vi "输入读取.vi"() -> (3 "输入读取":T1)   [LabVIEW 2017]
panel:
  in  "屏蔽光栅":bool
  out "运行时间":dbl
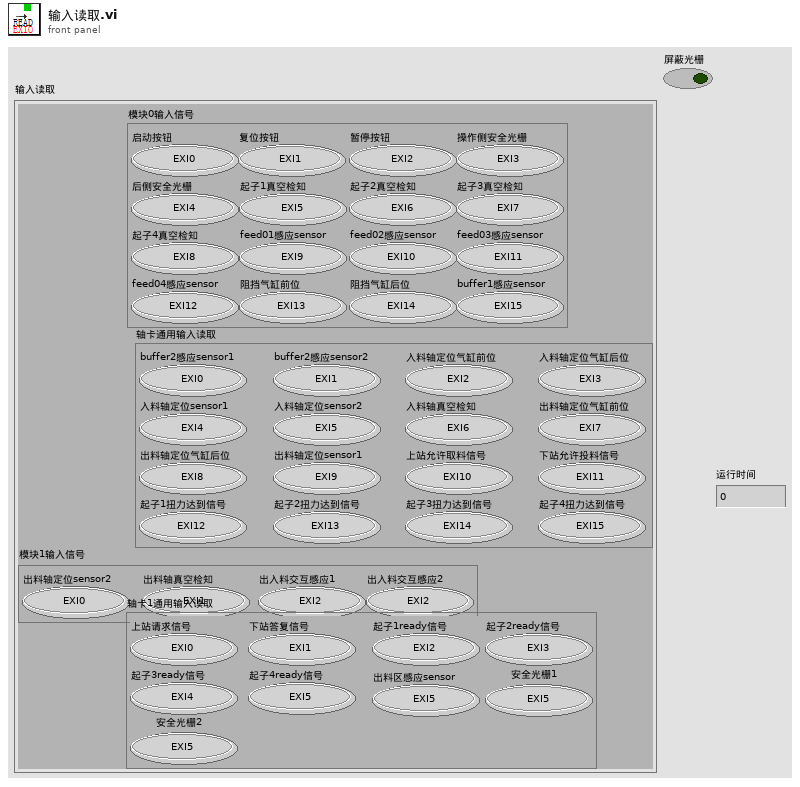
[diagram p1: front panel]
types:
  T1 = typedef "输入读取.ctl" = cluster{"模块0输入信号":T2, "轴卡通用输入读取":T3, "模块1输入信号":T4, "轴卡1通用输入读取":T5}
  T2 = typedef "模块0输入读取.ctl" = cluster{"启动按钮":bool, "复位按钮":bool, "暂停按钮":bool, "操作侧安全光栅":bool, "后侧安全光栅":bool, "起子1真空检知":bool, "起子2真空检知":bool, "起子3真空检知":bool, "起子4真空检知":bool, "feed01感应sensor":bool, "feed02感应sensor":bool, "feed03感应sensor":bool, "feed04感应sensor":bool, "阻挡气缸前位":bool, "阻挡气缸后位":bool, "buffer1感应sensor":bool}
  T3 = typedef "轴卡0通用输入读取.ctl" = cluster{"buffer2感应sensor1":bool, "buffer2感应sensor2":bool, "入料轴定位气缸前位":bool, "入料轴定位气缸后位":bool, "入料轴定位sensor1":bool, "入料轴定位sensor2":bool, "入料轴真空检知":bool, "出料轴定位气缸前位":bool, "出料轴定位气缸后位":bool, "出料轴定位sensor1":bool, "上站允许取料信号":bool, "下站允许投料信号":bool, "起子1扭力达到信号":bool, "起子2扭力达到信号":bool, "起子3扭力达到信号":bool, "起子4扭力达到信号":bool}
  T4 = typedef "模块1输入读取.ctl" = cluster{"出料轴定位sensor2":bool, "出料轴真空检知":bool, "出入料交互感应1":bool, "出入料交互感应2":bool}
  T5 = typedef "轴卡1通用输入读取.ctl" = cluster{"上站请求信号":bool, "下站答复信号":bool, "起子1ready信号":bool, "起子2ready信号":bool, "起子3ready信号":bool, "起子4ready信号":bool, "出料区感应sensor":bool, "安全光栅1":bool, "安全光栅2":bool}
  T6 = typedef "配置检索操作.ctl" = enum16{"配置检索", "名称提取", "寄存器提取"}
  T7 = typedef "输入&输出配置提取集合.ctl" = cluster{"IO配置名称":string[], "IO配置点位地址":string[], "IO配置名称索引":i32[], "取反信息":i32[], "簇属性集合":string[]}
  T8 = cluster{"[0]":bool, "[1]":bool, "[2]":bool, "[3]":bool, "[4]":bool, "[5]":bool, "[6]":bool, "[7]":bool, "[8]":bool, "[9]":bool, "[10]":bool, "[11]":bool, "[12]":bool, "[13]":bool, "[14]":bool, "[15]":bool}
  T9 = cluster{"[0]":bool, "[1]":bool, "[2]":bool, "[3]":bool}
  T10 = cluster{"[0]":bool, "[1]":bool, "[2]":bool, "[3]":bool, "[4]":bool, "[5]":bool, "[6]":bool, "[7]":bool, "[8]":bool}
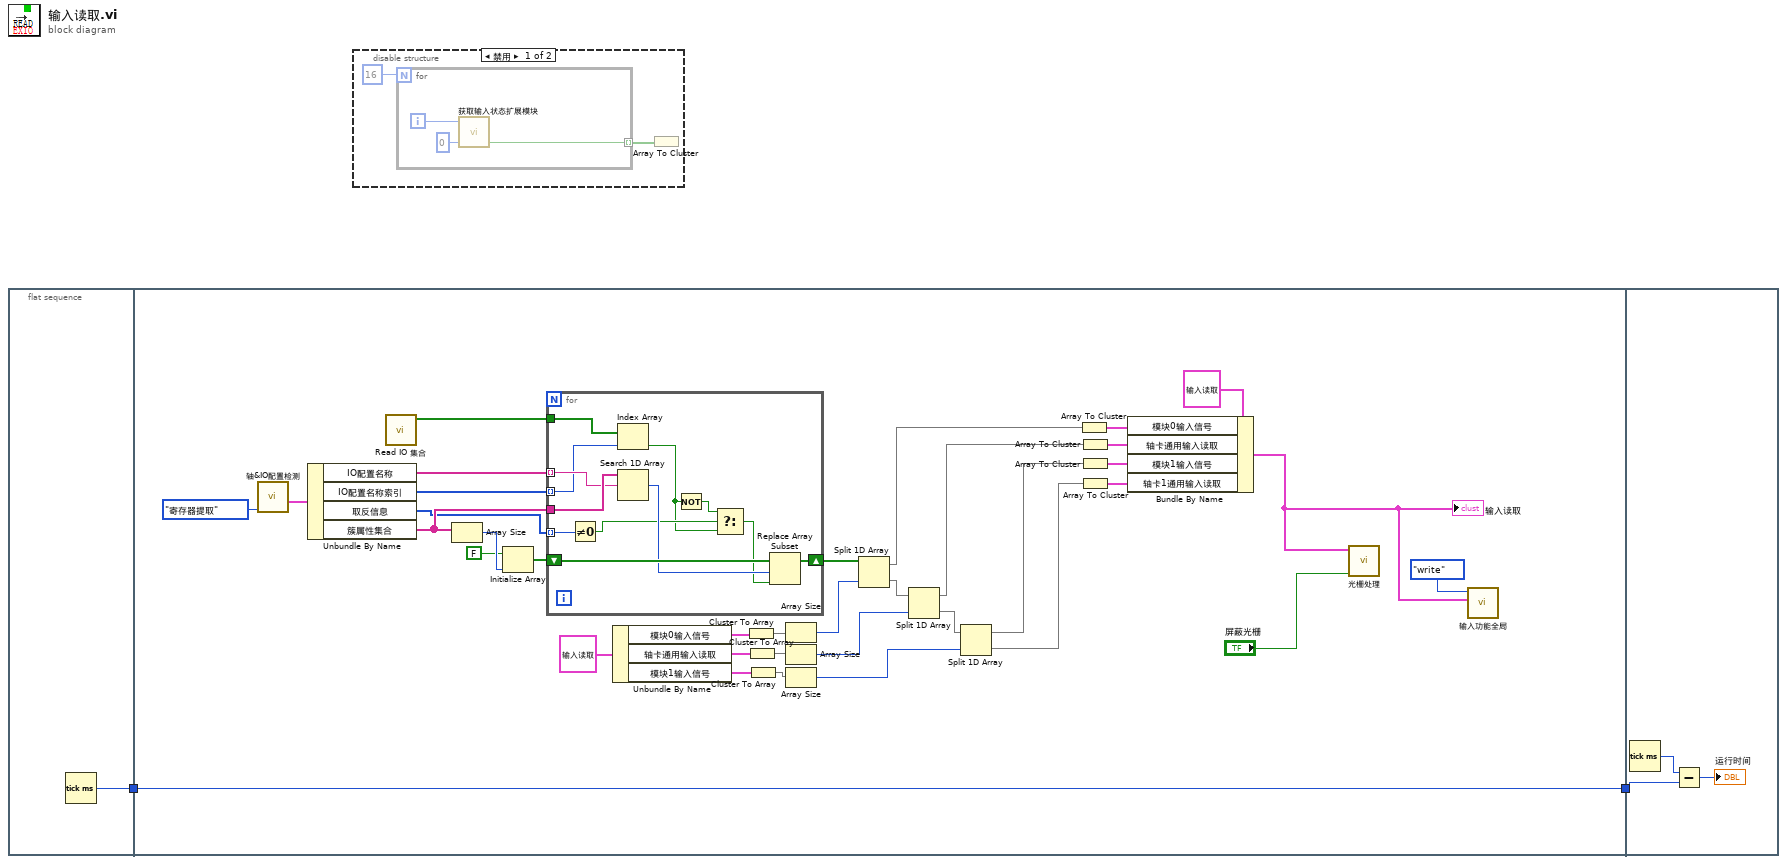
[diagram p0: block diagram]
diagram:
  n1 = flat-sequence {
    tunnel: [w3] -> w1
    tunnel: [w9] -> w2
    tunnel: w1 -> [w9]
    tunnel: w2 -> [w52]
    frame #0 {
      n2 = Tick Count (ms)() -> (millisecond timer value=w3:u32)
    }
    frame #1 {
      n3 = call "轴&IO配置检测.vi"("配置检索操作"=配置检索操作."寄存器提取") -> ("输入配置提取集合"=w37:T7)  [unwired: 7 in, 3 out]
      n4 = Unbundle By Name(w37) -> ("IO配置名称"=w34:string[], "IO配置名称索引"=w32:i32[], "取反信息"=w8:i32[], "簇属性集合"=w33:string[])
      n5 = call "Read IO 集合.vi"() -> ("IO集合"=w31:bool[])  [unwired: 11 in]
      n6 = Array Size(array=w33) -> (size(s)=w36:i32)
      n7 = Initialize Array(FALSE, w36) -> (w30:bool[])
      n8 = for {
        tunnel: w34 -> [w50] mode=indexing
        tunnel: w33 -> [w51]
        tunnel: w32 -> [w48] mode=indexing
        tunnel: w31 -> [w49]
        shift-right: [w45] -> w22
        shift-left: w30 -> [w47]
        tunnel: w8 -> [w44] mode=indexing
        n9 = Not Equal To 0?(x=w44) -> (x != 0?=w43:bool)
        n10 = Index Array(array=w49, index=w48) -> (element=w41:bool)
        n11 = Search 1D Array(1D array=w51, element=w50) -> (index of element=w46:i32)  [unwired: 1 in]
        n12 = Not(x=w41) -> (.not. x?=w42:bool)
        n13 = Select(t=w42, s=w43, f=w41) -> (s? t:f=w40:bool)
        n14 = Replace Array Subset(array=w47, new element=w40, index=w46) -> (w45:bool[])
      }
      n15 = Unbundle By Name(T1 {"模块0输入信号"={"启动按钮"=FALSE, "复位按钮"=FALSE, "暂停按钮"=FALSE, "操作侧安全光栅"=FALSE, "后侧安全光栅"=FALSE, "起子1真空检知"=FALSE, "起子2真空检知"=FALSE, "起子3真空检知"=FALSE, "起子4真空检知"=FALSE, "feed01感应sensor"=FALSE, "feed02感应sensor"=FALSE, "feed03感应sensor"=FALSE, "feed04感应sensor"=FALSE, "阻挡气缸前位"=FALSE, "阻挡气缸后位"=FALSE, "buffer1感应sensor"=FALSE}, "轴卡通用输入读取"={"buffer2感应sensor1"=FALSE, "buffer2感应sensor2"=FALSE, "入料轴定位气缸前位"=FALSE, "入料轴定位气缸后位"=FALSE, "入料轴定位sensor1"=FALSE, "入料轴定位sensor2"=FALSE, "入料轴真空检知"=FALSE, "出料轴定位气缸前位"=FALSE, "出料轴定位气缸后位"=FALSE, "出料轴定位sensor1"=FALSE, "上站允许取料信号"=FALSE, "下站允许投料信号"=FALSE, "起子1扭力达到信号"=FALSE, "起子2扭力达到信号"=FALSE, "起子3扭力达到信号"=FALSE, "起子4扭力达到信号"=FALSE}, "模块1输入信号"={"出料轴定位sensor2"=FALSE, "出料轴真空检知"=FALSE, "出入料交互感应1"=FALSE, "出入料交互感应2"=FALSE}, "轴卡1通用输入读取"={"上站请求信号"=FALSE, "下站答复信号"=FALSE, "起子1ready信号"=FALSE, "起子2ready信号"=FALSE, "起子3ready信号"=FALSE, "起子4ready信号"=FALSE, "出料区感应sensor"=FALSE, "安全光栅1"=FALSE, "安全光栅2"=FALSE}} ("输入读取")) -> ("模块0输入信号"=w28:T2, "轴卡通用输入读取"=w27:T3, "模块1输入信号"=w26:T4)
      n16 = Cluster To Array(cluster=w28) -> (array=w25:bool[])
      n17 = Cluster To Array(cluster=w27) -> (array=w24:bool[])
      n18 = Cluster To Array(cluster=w26) -> (array=w23:bool[])
      n19 = Array Size(array=w25) -> (size(s)=w21:i32)
      n20 = Array Size(array=w24) -> (size(s)=w19:i32)
      n21 = Array Size(array=w23) -> (size(s)=w17:i32)
      n22 = Split 1D Array(array=w22, index=w21) -> (first subarray=w16:bool[], second subarray=w20:bool[])
      n23 = Split 1D Array(array=w20, index=w19) -> (first subarray=w14:bool[], second subarray=w18:bool[])
      n24 = Split 1D Array(array=w18, index=w17) -> (first subarray=w12:bool[], second subarray=w10:bool[])
      n25 = Array To Cluster(array=w16) -> (cluster=w15:T8)
      n26 = Array To Cluster(array=w14) -> (cluster=w13:T8)
      n27 = Array To Cluster(array=w12) -> (cluster=w11:T9)
      n28 = Array To Cluster(array=w10) -> (cluster=w7:T10)
      n29 = Bundle By Name(cluster=T1 {"模块0输入信号"={"启动按钮"=FALSE, "复位按钮"=FALSE, "暂停按钮"=FALSE, "操作侧安全光栅"=FALSE, "后侧安全光栅"=FALSE, "起子1真空检知"=FALSE, "起子2真空检知"=FALSE, "起子3真空检知"=FALSE, "起子4真空检知"=FALSE, "feed01感应sensor"=FALSE, "feed02感应sensor"=FALSE, "feed03感应sensor"=FALSE, "feed04感应sensor"=FALSE, "阻挡气缸前位"=FALSE, "阻挡气缸后位"=FALSE, "buffer1感应sensor"=FALSE}, "轴卡通用输入读取"={"buffer2感应sensor1"=FALSE, "buffer2感应sensor2"=FALSE, "入料轴定位气缸前位"=FALSE, "入料轴定位气缸后位"=FALSE, "入料轴定位sensor1"=FALSE, "入料轴定位sensor2"=FALSE, "入料轴真空检知"=FALSE, "出料轴定位气缸前位"=FALSE, "出料轴定位气缸后位"=FALSE, "出料轴定位sensor1"=FALSE, "上站允许取料信号"=FALSE, "下站允许投料信号"=FALSE, "起子1扭力达到信号"=FALSE, "起子2扭力达到信号"=FALSE, "起子3扭力达到信号"=FALSE, "起子4扭力达到信号"=FALSE}, "模块1输入信号"={"出料轴定位sensor2"=FALSE, "出料轴真空检知"=FALSE, "出入料交互感应1"=FALSE, "出入料交互感应2"=FALSE}, "轴卡1通用输入读取"={"上站请求信号"=FALSE, "下站答复信号"=FALSE, "起子1ready信号"=FALSE, "起子2ready信号"=FALSE, "起子3ready信号"=FALSE, "起子4ready信号"=FALSE, "出料区感应sensor"=FALSE, "安全光栅1"=FALSE, "安全光栅2"=FALSE}} ("输入读取"), "模块0输入信号"=w15, "轴卡通用输入读取"=w13, "模块1输入信号"=w11, "轴卡1通用输入读取"=w7) -> (w5:T1)
      "输入读取" <- w5
      n30 = call "光栅处理.vi"("屏蔽光栅"="屏蔽光栅", "输入读取"=w5) -> ()  [unwired: 10 in]
      n31 = call "输入功能全局.vi"("输入"=w5, "选项"=enum16{"initialize", "read", "write"}."write") -> ()  [unwired: 9 in, 1 out]
    }
    frame #2 {
      n32 = Tick Count (ms)() -> (millisecond timer value=w54:u32)
      n33 = Subtract(x=w54, y=w52) -> (x-y=→"运行时间":u32)
    }
  }
  n34 = disable-structure shown="禁用" {
    frame Disabled {
      n35 = for {
        N: 16 -> [_]
        tunnel: [w57] -> w55 mode=indexing
        i -> [w58]
        n36 = call "获取输入状态扩展模块.vi"("mdl"=i16 0, "端口号"=w58) -> ("读取状态"=w57:bool)  [unwired: 2 in, 1 out]
      }
      n37 = Array To Cluster(array=w55) -> ()  [unwired: 1 out]
    }
    frame Enabled {
    }
  }
